vi "clear Session Data.vi"(0 "OBJ - Measurement Session in":refnum<class "Text Device Session.lvclass">, 11 "error in":errorcluster) -> (4 "OBJ - Measurement Session out":refnum<class "Text Device Session.lvclass">, 15 "error out":errorcluster)   [LabVIEW 2015, in "Text Device Session.lvclass"]
doc: "OVERRIDE VI\nPlaceholder for decendant classes to clear session information and close references."
uses:
  Text Device Session.lvclass
  File Access/Config Data/Config Data.lvclass
  Session Log/System Log.lvclass
  Text Device Session.lvclass/Text Device Session.ctl
  <userlib>/_Session Fwk/Session - Root.lvclass
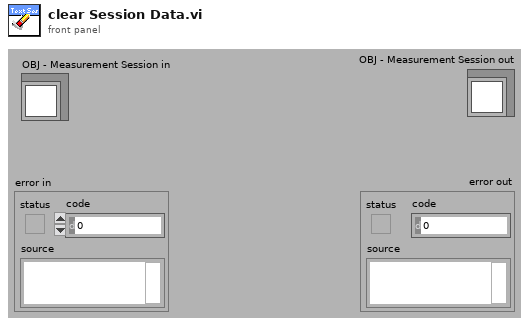
[diagram p1: front panel]
types:
  T1 = typedef "Session - Root.lvclass/Session Handle.ctl" = refnum<data-value>
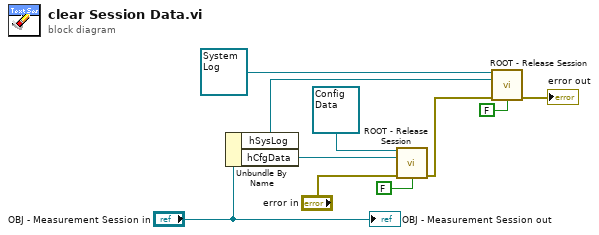
[diagram p0: block diagram]
diagram:
  n1 = Unbundle By Name("OBJ - Measurement Session in") -> ("hSysLog"=w6:T1, "hCfgData"=w9:T1)
  n2 = call <userlib>:"ROOT - Release Session.vi"("OBJ - Session in"=refnum<class "Config Data.lvclass"> refnum ("Config Data"), "Session Handle in"=w9, "error in (no error)"="error in", "force destroy? (F)"=FALSE) -> ("error out"=w2:errorcluster)  [unwired: 10 in, 1 out]
  n3 = call <userlib>:"ROOT - Release Session.vi"("OBJ - Session in"=refnum<class "System Log.lvclass"> refnum ("Sys Log"), "Session Handle in"=w6, "error in (no error)"=w2, "force destroy? (F)"=FALSE) -> ("error out"=→"error out":errorcluster)  [unwired: 10 in, 1 out]
  "OBJ - Measurement Session out" <- "OBJ - Measurement Session in"
